vi "Get dt.vi"(8 "error in (no error)":errorcluster, 11 "tdms file":refnum<k34>) -> (0 "error out":errorcluster, 3 "tdms file out":refnum<k34>, 4 "dt":dbl)   [LabVIEW 2015, in "Exposure Process.lvlib"]
uses:
  Exposure Process.lvlib
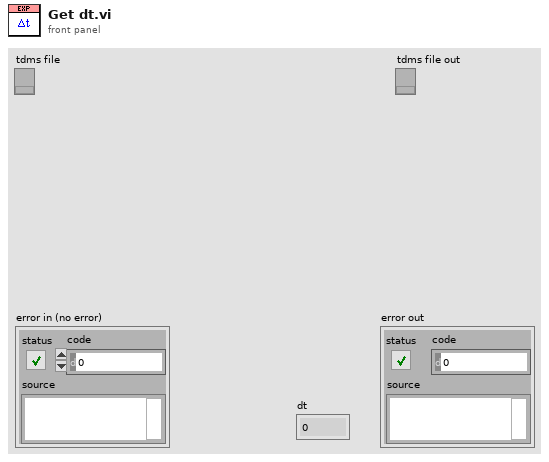
[diagram p1: front panel]
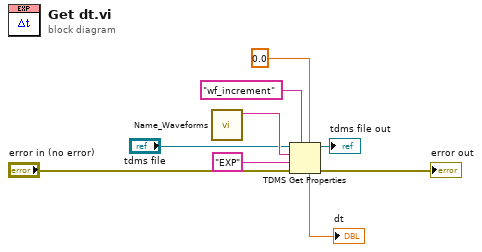
[diagram p0: block diagram]
diagram:
  n1 = call "Name_Waveforms.vi"() -> ("Name"=w9:string)  [unwired: 11 in]
  n2 = TDMS Get Properties(5:0.0, 7:"wf_increment" ("property name"), 8:"error in (no error)", 9:"EXP" ("channel name"), 10:w9, 11:"tdms file") -> (0:→"error out":errorcluster, 3:→"tdms file out":refnum<k34>, 4:→"dt":dbl)  [unwired: 3 out]
